vi "글로벌데이터.vi"() -> ()   [LabVIEW 2014]
panel:
  in  "숫자형":dbl
  out "불리언":bool
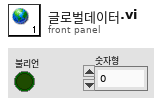
[diagram p1: front panel]
diagram:
